vi "Test Method Result Published.vi"(8 "error in (no error)":errorcluster, 11 "Result Observation Test In":refnum<class "Result Observation Test.lvclass">) -> (0 "error out":errorcluster, 3 "Result Observation Test Out":refnum<class "Result Observation Test.lvclass">)   [LabVIEW 2020, in "Result Observation Test.lvclass"]
uses:
  Result Observation Test.lvclass
  C:/Program Files (x86)/National Instruments/LabVIEW 2020/vi.lib/Astemes/LUnit/Test Case.lvclass
  LUnit Test Case Tests/LUnit Test Case V2 Test Double/Methods.ctl
  Result/Type.ctl
  <vilib>/Astemes/LUnit/Test Case.lvclass/Test Case.ctl
  <vilib>/Astemes/LUnit/Set Assertion Type.vi
  <vilib>/Astemes/LUnit/Palette/Pass.vi
  <vilib>/Astemes/LUnit/Palette/Fail.vi
  <vilib>/Astemes/LUnit/Add test result.vi
  <vilib>/Astemes/LUnit/LUnit Record Assertion Result.vi
  <vilib>/Astemes/LUnit/LUnit Aggregate Assertion Results.vi
  <vilib>/Astemes/LUnit/Method Result/LUnit Merge Status.vi
  <vilib>/Astemes/LUnit/LUnit Concatenate result strings.vi
  Mock Result Observer/Mock Result Observer.lvclass
  C:/Git/astemes-lunit/source/Rewrite Project/Result Observer/Result Observer.lvclass
  LUnit Test Case/LUnit Test Case V2.lvclass
  LUnit Test Case Tests/LUnit Test Case V2 Test Double/LUnit Test Case V2 Test Double.lvclass
  Result/Result.lvlib
  <vilib>/Astemes/LUnit/Test Case.lvclass
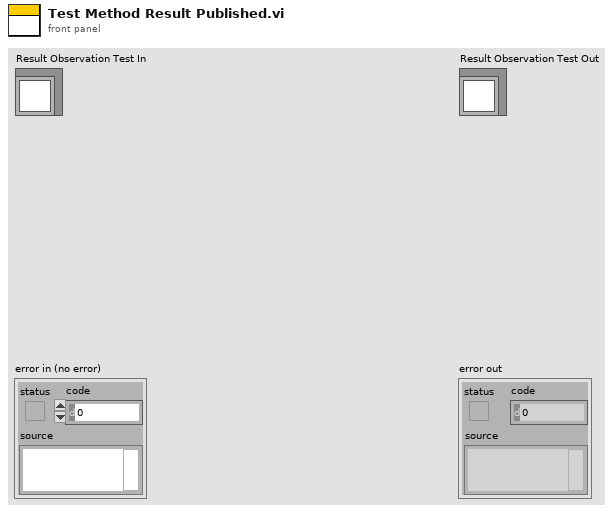
[diagram p1: front panel]
types:
  T1 = typedef "Result.lvlib/Type.ctl" = enum16{"Method", "Case", "Suite", "Pass", "Fail", "Skip", "Pass if", "Fail if", "Pass if Error", "Fail if Error", "Pass if Equal", "Fail if Equal"}
  T2 = typedef "LUnit Test Case V2 Test Double.lvclass/Methods.ctl" = enum16{"Test Failing Test.vi", "Test Passing Test.vi", "Test Error Test.vi", "Test Skip Test.vi", "Test Passing Pass If Test.vi", "Test Failing Pass If Test.vi", "Test Failing Fail If Test.vi", "Test Passing Fail If Test.vi", "Test Passing Pass If Error Test.vi", "Test Failing Pass If Error Test.vi", "Test Passing Fail If Error Test.vi", "Test Failing Fail If Error Test.vi", "Test Passing Pass If Equal Test.vi", "Test Failing Pass If Equal Test.vi", "Test Failing Fail If Equal Test.vi", "Test Passing Fail If Equal Test.vi"}
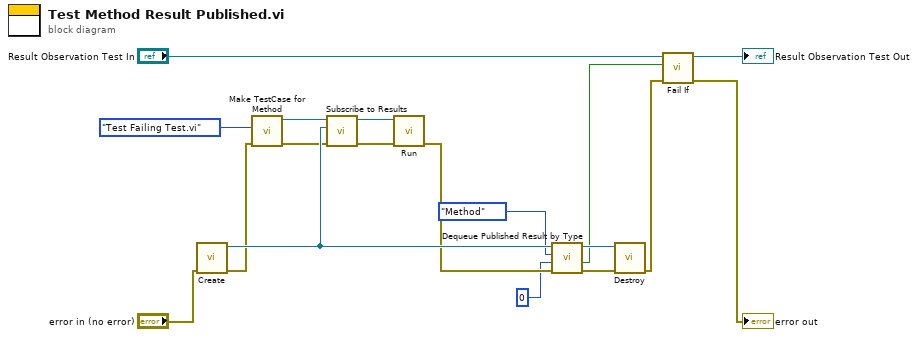
[diagram p0: block diagram]
diagram:
  n1 = call "Create.vi"("error in (no error)"="error in (no error)") -> ("error out"=w9:errorcluster, "Mock Result Observer out"=w12:refnum<class "Mock Result Observer.lvclass">)  [unwired: 9 in]
  n2 = call "Make TestCase for Method.vi"("error in (no error)"=w9, "Test Method"=Methods."Test Failing Test.vi") -> ("error out"=w8:errorcluster, "LUnit Test Case V2 out"=w13:refnum<class "LUnit Test Case V2.lvclass">)  [unwired: 8 in]
  n3 = call-dynamic "Subscribe to Results.vi"("error in (no error)"=w8, "Result Observer"=w12, "LUnit Test Case V2 In"=w13) -> ("error out"=w7:errorcluster, "LUnit Test Case V2 Out"=w11:refnum<class "LUnit Test Case V2.lvclass">)  [unwired: 7 in]
  n4 = call-dynamic "Run.vi"("error in (no error)"=w7, "LUnit Test Case V2 in"=w11) -> ("error out"=w6:errorcluster)  [unwired: 8 in, 1 out]
  n5 = call "Dequeue Published Result by Type.vi"("error in (no error)"=w6, "timeout in ms"=0 ("timeout in ms (-1)"), "Result Type"=Type."Method", "Mock Result Observer In"=w12) -> ("error out"=w16:errorcluster, "timed out?"=w3:bool, "Mock Result Observer Out"=w17:refnum<class "Mock Result Observer.lvclass">)  [unwired: 4 in, 1 out]
  n6 = call "Destroy.vi"("error in (no error)"=w16, "Mock Result Observer in"=w17) -> ("error out"=w2:errorcluster)  [unwired: 9 in]
  n7 = call <vilib>:"Fail If.vi"("error in (no error)"=w2, "Fail?"=w3, "LUnit Test Case In"="Result Observation Test In") -> ("error out"=→"error out":errorcluster, "LUnit Test Case Out"=→"Result Observation Test Out":refnum<class "Result Observation Test.lvclass">)  [unwired: 7 in]
